vi "KsPS_Control.vi"() -> ()   [LabVIEW 2015]
doc: "This VI tool is designed to control Agilent/Keysight N67xx series power supply mainframes.\n\nFor support contact: Aldrin Albano, J54147"
uses:
  <vilib>/Utility/sysdir.llb/System Directory Type.ctl
  <vilib>/Utility/file.llb/Read Delimited Spreadsheet (string).vi
  <vilib>/Utility/file.llb/Write Delimited Spreadsheet (string).vi
  <instrlib>/Agilent N6700 Series/Agilent N6700 Series.lvlib
panel:
  in  "Tab Control":enum32{"Main", "Config", "Status"}(tab)
  out "OVP1":dbl format="%.3f"
  out "OVP4":dbl format="%.3f"
  out "OVP3":dbl format="%.3f"
  out "OVP2":dbl format="%.3f"
  out "State":string="Close GUI"
  out "Revision":string
  out "Ch4-I":dbl format="%.3f"
  out "Ch4-V":dbl format="%.3f"
  out "Ch3-I":dbl format="%.3f"
  out "Ch3-V":dbl format="%.3f"
  out "Ch2-I":dbl format="%.3f"
  out "Ch2-V":dbl format="%.3f"
  out "Ch1-V":dbl format="%.3f"
  out "Ch1-I":dbl format="%.3f"
  in  "Auto On/Off":bool
  in  "Auto Query":bool
  in  "Lock":bool=TRUE
  in  "Rvs Pwr Down":bool=TRUE
  in  "On/Off":bool
  in  "PS Settings":string[][](table)
  in  "Config_PATH":path
  in  "Load":bool
  in  "Query":bool
  in  "Save":bool
  in  "ResetOVP":bool
  in  "Qry Intrvl (ms)":u32=5000
  out "Open VISA Sessions":refnum<visa-resource-name>[](array[refnum])
  out "INI PATH":path
  out "Error Out":errorcluster
  # "OVP"
  # "OVP"
  # "OVP"
  # "OVP"
  # "V"
  # "A"
  # "V"
  # "A"
  # "V"
  # "A"
  # "V"
  # "A"
  # "Keysight N6700 Series PS Control Utility"
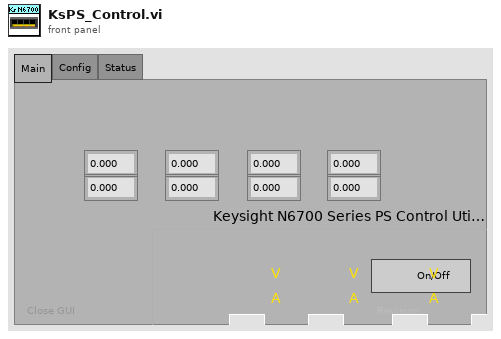
[diagram p1: front panel]
types:
  T1 = cluster{"PS Settings":string[][], "Config_PATH":path, "INI_PATH":path, "Open Sessions":refnum<visa-resource-name>[], "This VI":refnum<vi>, "VI Name":string}
  T2 = typedef "System Directory Type.ctl" = i32
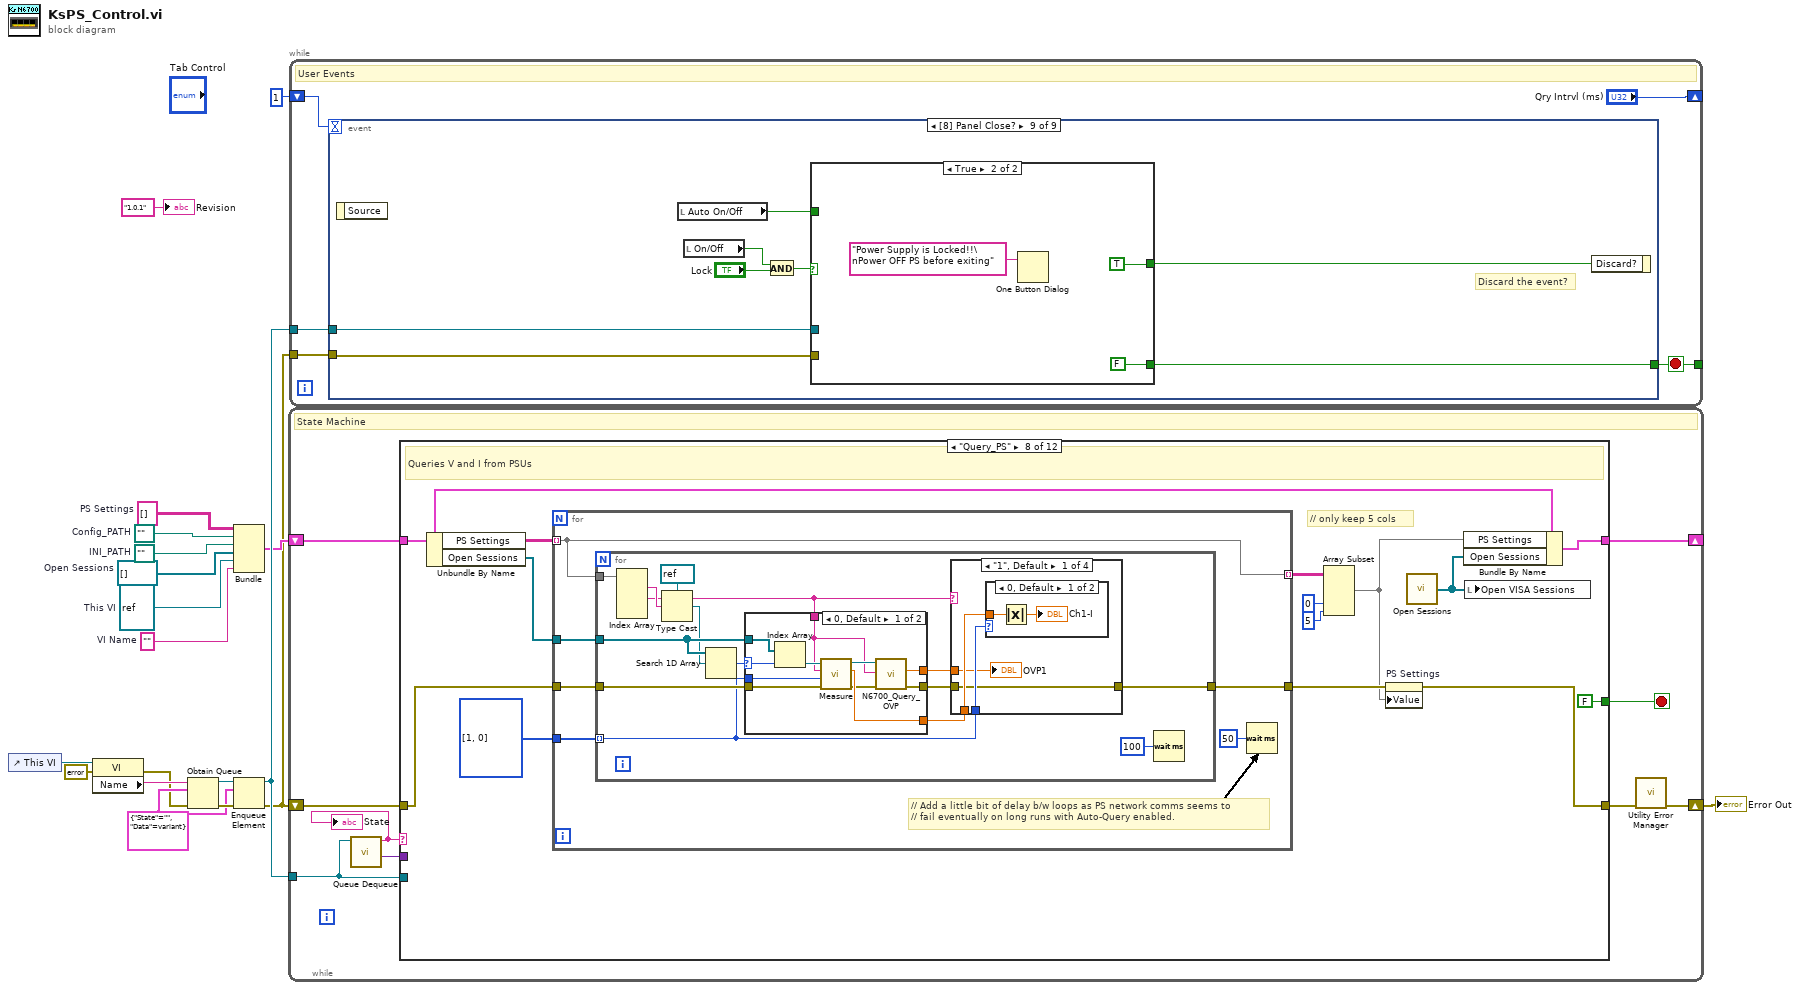
[diagram p0: block diagram]
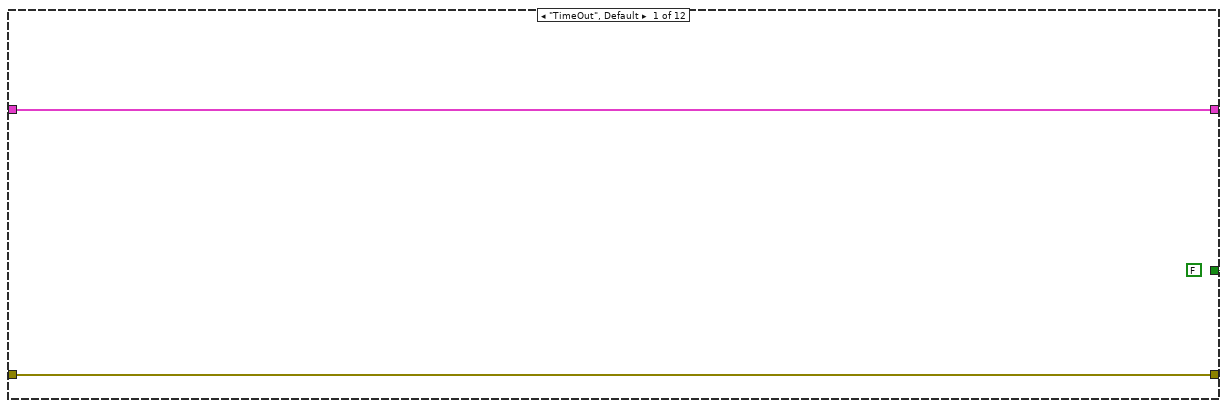
[diagram p2: hidden frame]
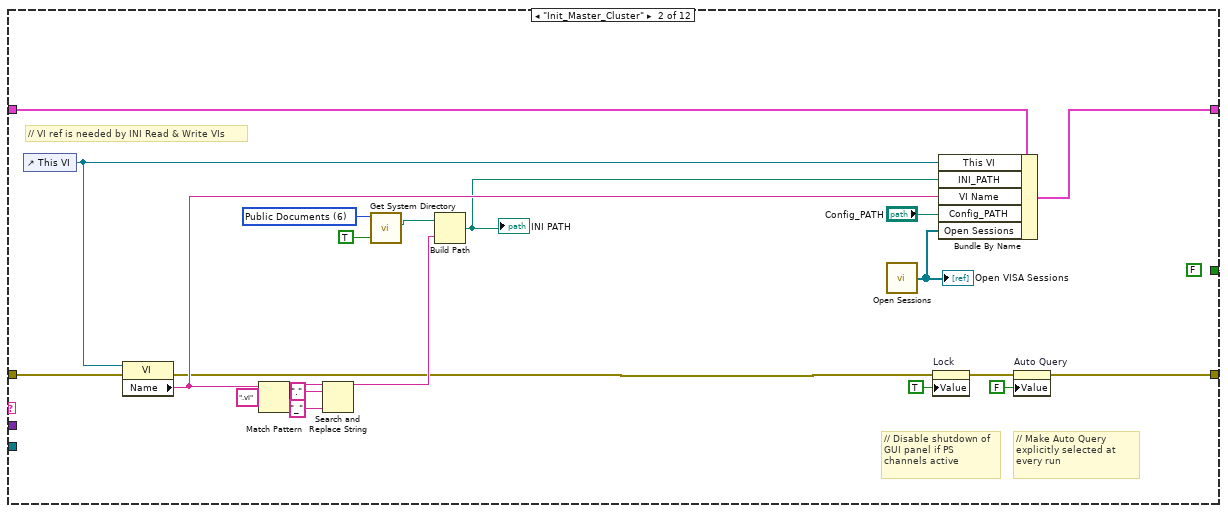
[diagram p3: hidden frame]
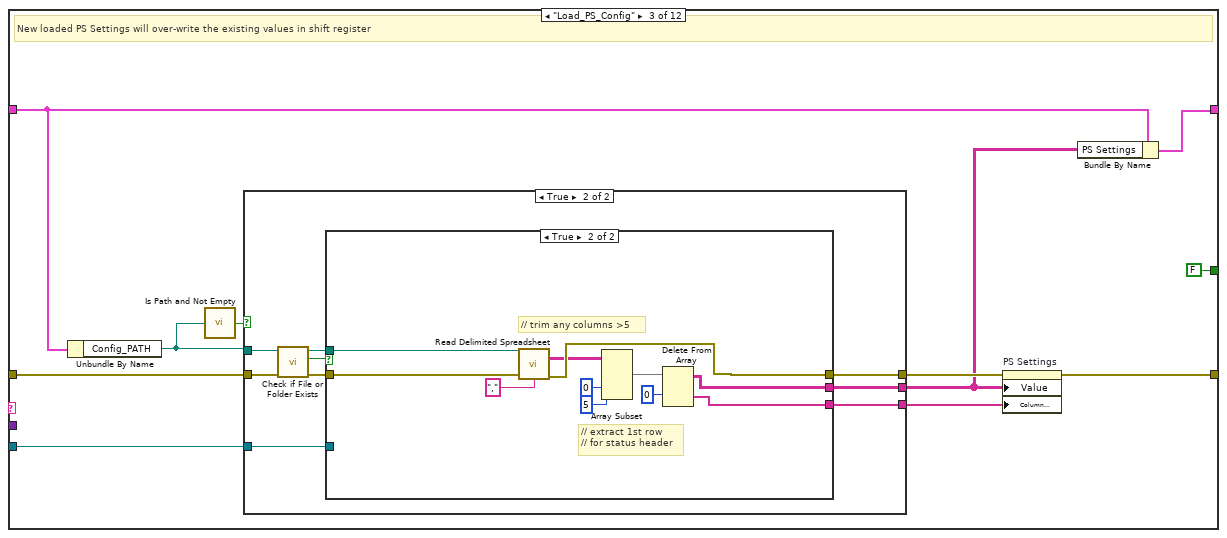
[diagram p4: hidden frame]
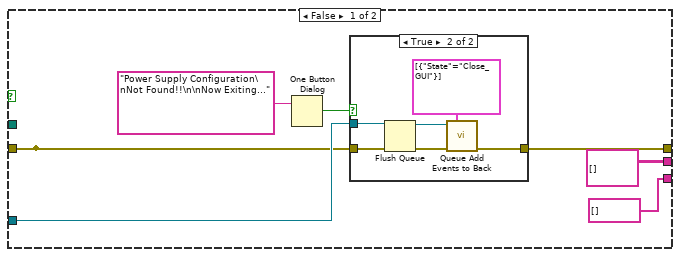
[diagram p5: hidden frame]
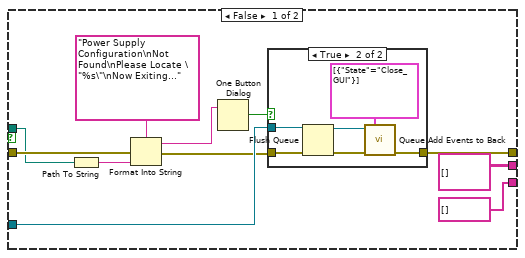
[diagram p7: hidden frame]
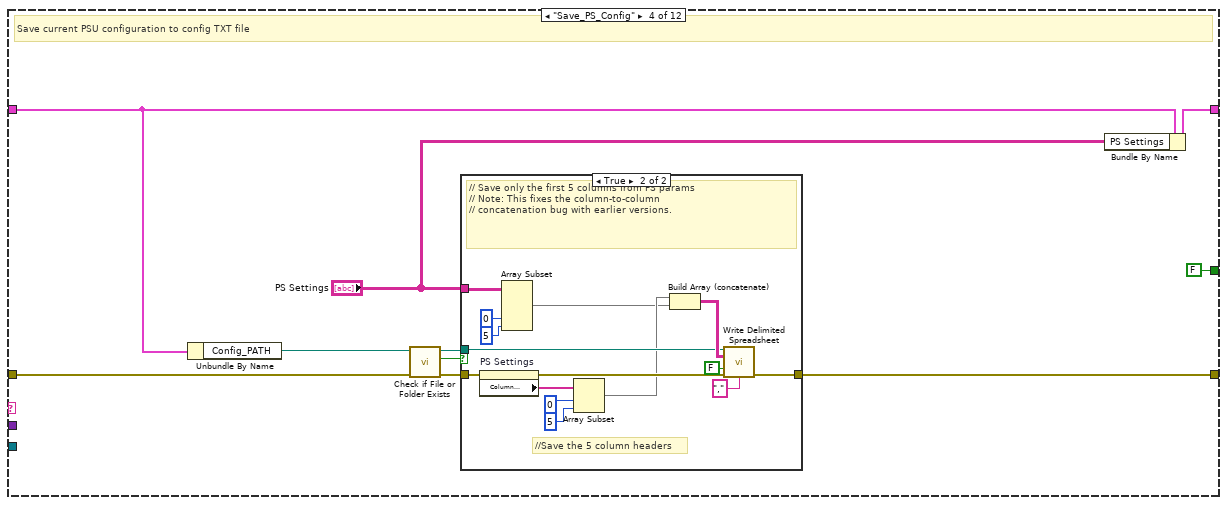
[diagram p9: hidden frame]
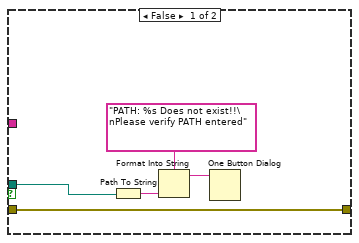
[diagram p10: hidden frame]
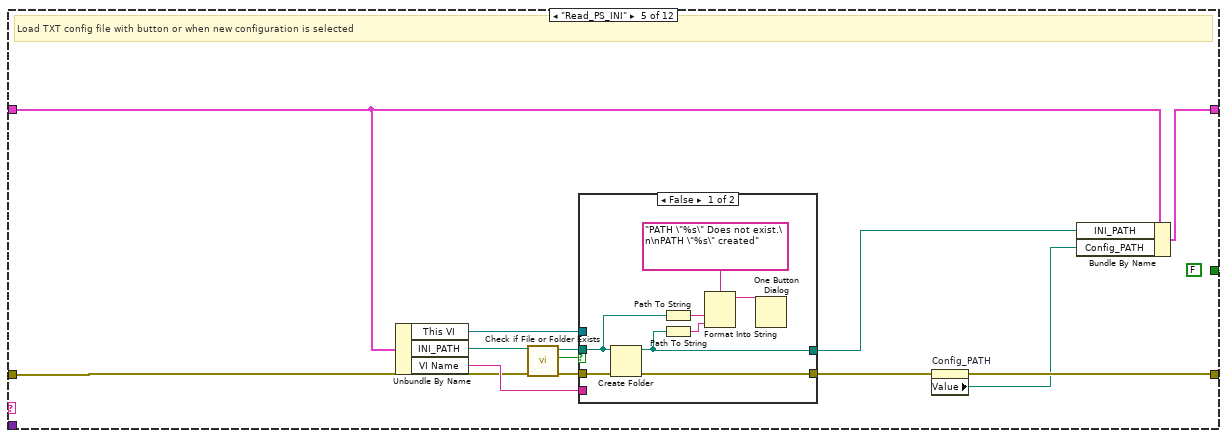
[diagram p11: hidden frame]
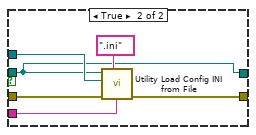
[diagram p12: hidden frame]
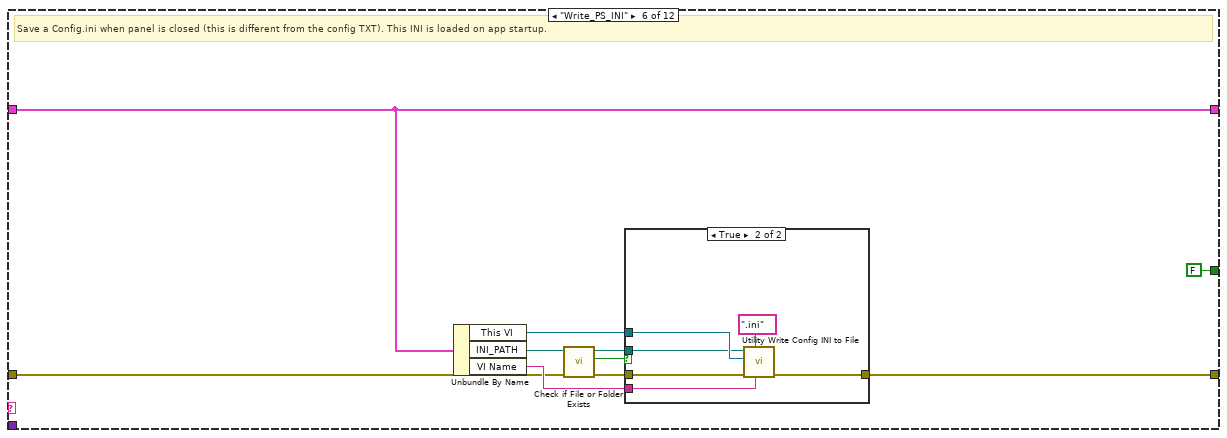
[diagram p13: hidden frame]
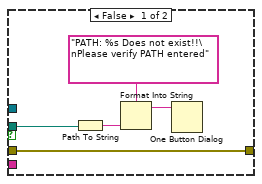
[diagram p14: hidden frame]
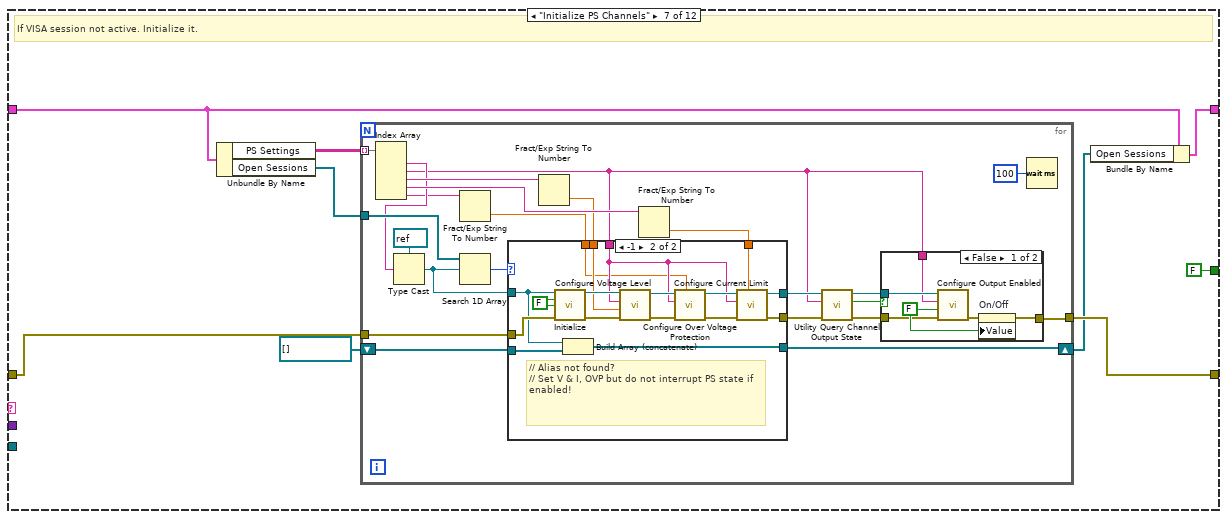
[diagram p15: hidden frame]
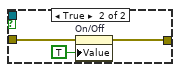
[diagram p16: hidden frame]
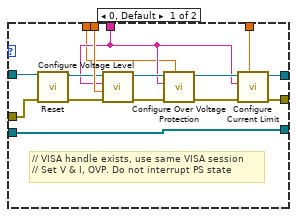
[diagram p17: hidden frame]
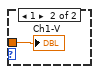
[diagram p18: hidden frame]
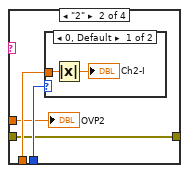
[diagram p19: hidden frame]
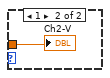
[diagram p20: hidden frame]
diagram:
  w2 = ""  # VI Name
  w3 = refnum<visa-resource-name>[] []  # Open Sessions
  w4 = refnum<vi> refnum  # This VI
  w6 = string[][] []  # PS Settings
  w7 = path ""  # INI_PATH
  w8 = path ""  # Config_PATH
  w17 = cluster{"State":string, "Data":variant} {"State"="", "Data"=variant} ("Cluster")
  n1 = control-ref of="This VI"() -> (w1:refnum<vi>)
  n2 = property class="VI"(reference=w1, error in=errorcluster {"status"=FALSE, "code"=0, "source"=""} ("Error In")) -> (error out=w13:errorcluster, "Name"=w15:string)  [unwired: 1 out]
  n3 = Obtain Queue(name (unnamed)=w15, element data type=w17, error in (no error)=w13) -> (queue out=w18:refnum<queue>, error out=w19:errorcluster)  [unwired: 2 in, 1 out]
  n4 = Bundle("PS Settings"=w6, "Config_PATH"=w8, "INI_PATH"=w7, "Open Sessions"=w3, "This VI"=w4, "VI Name"=w2) -> (w9:T1)  [unwired: 1 in]
  n5 = Enqueue Element(queue=w18, element=w17, error in (no error)=w19) -> (queue out=w16:refnum<queue>, error out=w5:errorcluster)  [unwired: 1 in, 1 out]
  n6 = while {
    shift-right: [w28] -> w11
    shift-left: w5 -> [w25]
    shift-right: [w20] -> _
    shift-left: w9 -> [w24]
    tunnel: w16 -> [w21]
    stop <- w26 stop-if-true
    # "State Machine"
    n7 = call "Queue Dequeue.vi"("Queue In"=w21) -> ("Data"=w22:variant, "State"=w23:string)  [unwired: 8 in, 1 out]
    "State" <- w23
    n8 = case shown="\"Query_PS\"" w23 {
      tunnel: w25 -> [w30 w52 w59 w123 w155 w178 w196 w279 w342 w361 w377 w395]
      tunnel: [w30 w47 w56 w124 w147 w182 w201 w276 w345 w357 w380 w390] -> w27
      tunnel: w21 -> [_ _ w58 _ _ _ _ _ _ _ _ w397]
      tunnel: [FALSE FALSE FALSE FALSE FALSE FALSE FALSE FALSE FALSE FALSE FALSE TRUE] -> w26
      tunnel: w24 -> [w29 w50 w55 w117 w158 w180 w199 w278 w343 w356 w378 w393]
      tunnel: w22 -> [_ _ _ _ _ _ _ _ _ _ _ _]
      tunnel: [w29 w51 w61 w122 w157 w180 w198 w271 w343 w356 w378 w393] -> w20
      frame "TimeOut", Default {
        (unwired) FALSE
      }
      frame "Init_Master_Cluster" {
        w43 = T2 6 items=["User Home"=0, "User Desktop"=1, "User Documents"=2, "User Application Data"=3, "User Preferences"=4, "User Temporary"=5, "Public Documents"=6, "Public Application Data"=7, "Public Preferences"=8, "Public Cache"=13, "System Core Libraries"=9, "System Installed Libraries"=10, "Application Files"=11, "Boot Volume Root"=12] ("system directory type")
        (unwired) FALSE
        # "// Disable shutdown of GUI panel if PS channels active"
        # "// Make Auto Query explicitly selected at every run"
        # "// VI ref is needed by INI Read & Write VIs"
        n9 = control-ref of="This VI"() -> (w48:refnum<vi>)
        n10 = property class="VI"(reference=w48, error in=w52) -> (error out=w33:errorcluster, "Name"=w35:string)  [unwired: 1 out]
        n11 = Match Pattern(string=w35, regular expression=".vi") -> (before substring=w37:string)  [unwired: 1 in, 3 out]
        n12 = Search and Replace String(input string=w37, search string=".", replace string="_" ("replace string (\"\")")) -> (result string=w36:string)  [unwired: 5 in, 3 out]
        n13 = call <vilib>:"Get System Directory.vi"("create directory if not found? (F)"=TRUE, "system directory type"=w43) -> ("system directory"=w41:path)  [unwired: 9 in]
        n14 = Build Path(base path=w41, name or relative path=w36) -> (appended path=w34:path)
        "INI PATH" <- w34
        n15 = call <vilib>:"Open Sessions.vi"() -> ("Array of Refnums"=w49:refnum<visa-resource-name>[])  [unwired: 2 in]
        "Open VISA Sessions" <- w49
        n16 = property on="Lock" class="Bool (strict)"(error in=w33, "Value"=TRUE ("Lock")) -> (error out=w45:errorcluster)  [unwired: 1 in, 1 out]
        n17 = Bundle By Name(cluster=w50, "This VI"=w48, "INI_PATH"=w34, "VI Name"=w35, "Config_PATH"="Config_PATH", "Open Sessions"=w49) -> (w51:T1)
        n18 = property on="Auto Query" class="Bool (strict)"(error in=w45, "Value"=FALSE ("Auto Query")) -> (error out=w47:errorcluster)  [unwired: 1 in, 1 out]
      }
      frame "Load_PS_Config" {
        # "New loaded PS Settings will over-write the existing values in shift register"
        n19 = Unbundle By Name(w55) -> ("Config_PATH"=w54:path)
        n20 = call <vilib>:"Is Path and Not Empty.vi"("path"=w54) -> ("Is Path and Not Empty?"=w57:bool)  [unwired: 4 in]
        n21 = case shown="True" w57 {
          tunnel: [w66 w86] -> w64
          tunnel: [string[] [] ("all rows") w85] -> w63
          tunnel: [string[][] [] w84] -> w60
          tunnel: w58 -> [w68 w83]
          tunnel: w59 -> [w66 w81]
          tunnel: w54 -> [_ w78]
          frame False {
            n22 = One Button Dialog(message="Power Supply Configuration\nNot Found!!\n\nNow Exiting...") -> (true=w67:bool)  [unwired: 1 in]
            n23 = case shown="True" w67 {
              tunnel: w68 -> [_ w75]
              tunnel: w66 -> [w71 w73]
              tunnel: [w71 w76] -> _
              frame False {
              }
              frame True {
                n24 = Flush Queue(queue=w75, error in (no error)=w73) -> (queue out=w74:refnum<queue>, error out=w72:errorcluster)  [unwired: 1 out]
                n25 = call "Queue Add Events to Back.vi"("Queue In"=w74, "State Array"=cluster{"State":string}[] [{"State"="Close_GUI"}], "Error In"=w72) -> ("Error Out"=w76:errorcluster)  [unwired: 11 in, 1 out]
              }
            }
          }
          frame True {
            n26 = call <vilib>:"Check if File or Folder Exists.vi"("error in (no error)"=w81, "path"=w78) -> ("error out"=w80:errorcluster, "file or folder exists?"=w79:bool, "dup path"=w82:path)  [unwired: 7 in]
            n27 = case shown="True" w79 {
              tunnel: [w93 w115] -> w86
              tunnel: [string[] [] ("all rows") w114] -> w85
              tunnel: [string[][] [] w113] -> w84
              tunnel: w80 -> [w90 w112]
              tunnel: w82 -> [w88 w111]
              tunnel: w83 -> [w95 _]
              frame False {
                n28 = Path To String(path=w88) -> (string=w87:string)
                n29 = Format Into String(format string="Power Supply Configuration\nNot Found\nPlease Locate \"%s\"\nNow Exiting..." ("message"), error in=w90, w87) -> (resulting string=w91:string, error out=w89:errorcluster)  [unwired: 1 in]
                n30 = One Button Dialog(message=w91) -> (true=w94:bool)  [unwired: 1 in]
                n31 = case shown="True" w94 {
                  tunnel: w95 -> [_ w102]
                  tunnel: w89 -> [w98 w100]
                  tunnel: [w98 w103] -> w93
                  frame False {
                  }
                  frame True {
                    n32 = Flush Queue(queue=w102, error in (no error)=w100) -> (queue out=w101:refnum<queue>, error out=w99:errorcluster)  [unwired: 1 out]
                    n33 = call "Queue Add Events to Back.vi"("Queue In"=w101, "State Array"=cluster{"State":string}[] [{"State"="Close_GUI"}], "Error In"=w99) -> ("Error Out"=w103:errorcluster)  [unwired: 11 in, 1 out]
                  }
                }
              }
              frame True {
                # "// trim any columns >5"
                # "// extract 1st row\n// for status header"
                n34 = call-poly <vilib>:"Read Delimited Spreadsheet.vi"("file path (dialog if empty)"=w111, "error in (no error)"=w112, "delimiter (\\t)"="," ("delimiter (\\t)")) -> ("all rows"=w106:string[][], "error out"=w115:errorcluster)  [unwired: 7 in, 4 out]
                n35 = Array Subset(array=w106, index (col)=0 ("index"), length (col)=5 ("length")) -> (w105:string[][])  [unwired: 2 in]
                n36 = Delete From Array(array=w105, index (row)=0) -> (deleted portion=w114:string[], array with subset deleted=w113:string[][])  [unwired: 2 in]
              }
            }
          }
        }
        n37 = property on="PS Settings" class="Tbl (strict)"(error in=w64, "Value"=w60, "Column Headers[]"=w63) -> (error out=w56:errorcluster)  [unwired: 1 in, 1 out]
        n38 = Bundle By Name(cluster=w55, "PS Settings"=w60) -> (w61:T1)
      }
      frame "Save_PS_Config" {
        # "Save current PSU configuration to config TXT file"
        n39 = Unbundle By Name(w117) -> ("Config_PATH"=w116:path)
        n40 = call <vilib>:"Check if File or Folder Exists.vi"("error in (no error)"=w123, "path"=w116) -> ("error out"=w120:errorcluster, "file or folder exists?"=w118:bool, "dup path"=w119:path)  [unwired: 7 in]
        n41 = case shown="True" w118 {
          tunnel: [w130 w142] -> w124
          tunnel: "PS Settings" -> [_ w134]
          tunnel: w119 -> [w126 w140]
          tunnel: w120 -> [w130 w133]
          frame False {
            n42 = Path To String(path=w126) -> (string=w128:string)
            n43 = Format Into String(format string="PATH: %s Does not exist!!\nPlease verify PATH entered", w128) -> (resulting string=w127:string)  [unwired: 2 in, 1 out]
            n44 = One Button Dialog(message=w127) -> ()  [unwired: 1 in, 1 out]
          }
          frame True {
            # "//Save the 5 column headers"
            # "// Save only the first 5 columns from PS params\n// Note: This fixes the column-to-column\n// concatenation bug with earlier versions."
            n45 = property on="PS Settings" class="Tbl (strict)"(error in=w133) -> (error out=w143:errorcluster, "Column Headers[]"=w137:string[])  [unwired: 1 in, 1 out]
            n46 = Array Subset(array=w134, index (col)=0 ("index"), length (col)=5 ("length")) -> (w131:string[][])  [unwired: 2 in]
            n47 = Array Subset(array=w137, index=0, length=5) -> (w132:string[])
            n48 = Build Array (concatenate)(w132, w131) -> (w141:string[][])
            n49 = call-poly <vilib>:"Write Delimited Spreadsheet.vi"("file path (dialog if empty)"=w140, "2D data"=w141, "append to file? (F)"=FALSE, "error in (no error)"=w143, "delimiter (\\t)"="," ("delimiter (\\t)")) -> ("error out"=w142:errorcluster)  [unwired: 9 in, 1 out]
          }
        }
        n50 = Bundle By Name(cluster=w117, "PS Settings"="PS Settings") -> (w122:T1)
      }
      frame "Read_PS_INI" {
        (unwired) FALSE
        # "Load TXT config file with button or when new configuration is selected"
        n51 = Unbundle By Name(w158) -> ("This VI"=w150:refnum<vi>, "INI_PATH"=w153:path, "VI Name"=w156:string)
        n52 = call <vilib>:"Check if File or Folder Exists.vi"("error in (no error)"=w155, "path"=w153) -> ("error out"=w154:errorcluster, "file or folder exists?"=w151:bool, "dup path"=w152:path)  [unwired: 7 in]
        n53 = case shown="False" w151 {
          tunnel: [w164 w171] -> w148
          tunnel: w154 -> [w164 w170]
          tunnel: w152 -> [w162 w167]
          tunnel: w150 -> [_ w169]
          tunnel: [w160 w167] -> w149
          tunnel: w156 -> [_ w168]
          frame False {
            n54 = Create Folder(path (use dialog)=w162, error in=w164) -> (created path=w160:path)  [unwired: 1 in, 2 out]
            n55 = Path To String(path=w162) -> (string=w163:string)
            n56 = Path To String(path=w160) -> (string=w161:string)
            n57 = Format Into String(format string="PATH \"%s\" Does not exist.\n\nPATH \"%s\" created", w163, w161) -> (resulting string=w165:string)  [unwired: 2 in, 1 out]
            n58 = One Button Dialog(message=w165) -> ()  [unwired: 1 in, 1 out]
          }
          frame True {
            n59 = call "Utility Load Config INI from File.vi"("File Name"=w168, "File Type"=".ini", "Error In"=w170, "reference"=w169, "Path In"=w167) -> ("Error Out"=w171:errorcluster)  [unwired: 5 in, 1 out]
          }
        }
        n60 = property on="Config_PATH" class="Path"(error in=w148) -> (error out=w147:errorcluster, "Value"=w146:path)  [unwired: 1 in, 1 out]
        n61 = Bundle By Name(cluster=w158, "INI_PATH"=w149, "Config_PATH"=w146) -> (w157:T1)
      }
      frame "Write_PS_INI" {
        # "Save a Config.ini when panel is closed (this is different from the config TXT). This INI is loaded on app startup."
        n62 = Unbundle By Name(w180) -> ("This VI"=w173:refnum<vi>, "INI_PATH"=w175:path, "VI Name"=w179:string)
        n63 = call <vilib>:"Check if File or Folder Exists.vi"("error in (no error)"=w178, "path"=w175) -> ("error out"=w177:errorcluster, "file or folder exists?"=w176:bool, "dup path"=w174:path)  [unwired: 7 in]
        n64 = case shown="True" w176 {
          tunnel: w177 -> [w187 w193]
          tunnel: [w187 w192] -> w182
          tunnel: w174 -> [w183 w188]
          tunnel: w173 -> [_ w190]
          tunnel: w179 -> [_ w189]
          frame False {
            n65 = Path To String(path=w183) -> (string=w185:string)
            n66 = Format Into String(format string="PATH: %s Does not exist!!\nPlease verify PATH entered", w185) -> (resulting string=w184:string)  [unwired: 2 in, 1 out]
            n67 = One Button Dialog(message=w184) -> ()  [unwired: 1 in, 1 out]
          }
          frame True {
            n68 = call "Utility Write Config INI to File.vi"("File Name"=w189, "File Type"=".ini", "Error In"=w193, "reference"=w190, "Path In"=w188) -> ("Error Out"=w192:errorcluster)  [unwired: 5 in, 1 out]
          }
        }
      }
      frame "Initialize PS Channels" {
        # "If VISA session not active. Initialize it."
        n69 = Unbundle By Name(w199) -> ("PS Settings"=w202:string[][], "Open Sessions"=w194:refnum<visa-resource-name>[])
        n70 = for {
          tunnel: w202 -> [w224] mode=indexing
          shift-right: [w222] -> w197
          shift-left: refnum<visa-resource-name>[] [] -> [w225]
          tunnel: [w208] -> w201
          tunnel: w196 -> [w216]
          tunnel: w194 -> [w215]
          n71 = Index Array(array=w224) -> (element #1=w214:string, element #2=w206:string, element #3=w220:string, element #4=w219:string, element #5=w204:string)  [unwired: 5 in]
          n72 = Type Cast(type=refnum<visa-resource-name> refnum ("VISA resource name"), x=w214) -> (*(type *) &x=w212:refnum<visa-resource-name>)
          n73 = Fract/Exp String To Number(string=w204) -> (number=w203:dbl)  [unwired: 3 in, 1 out]
          n74 = Search 1D Array(1D array=w215, element=w212) -> (index of element=w221:i32)  [unwired: 1 in]
          n75 = Fract/Exp String To Number(string=w220) -> (number=w217:dbl)  [unwired: 3 in, 1 out]
          n76 = Fract/Exp String To Number(string=w219) -> (number=w218:dbl)  [unwired: 3 in, 1 out]
          n77 = case shown="-1" w221 {
            tunnel: [w249 w266] -> w222
            tunnel: w225 -> [w249 w265]
            tunnel: [w247 w252] -> w210
            tunnel: w216 -> [w238 w264]
            tunnel: w212 -> [w240 w260]
            tunnel: w218 -> [w248 w261]
            tunnel: w217 -> [w242 w254]
            tunnel: w206 -> [w236 w253]
            tunnel: [w241 w251] -> w211
            tunnel: w203 -> [w235 w250]
            frame 0, Default {
              # "// VISA handle exists, use same VISA session\n// Set V & I, OVP. Do not interrupt PS state"
              n78 = call <instrlib>:"Reset.vi"("VISA resource name"=w240, "error in (no error)"=w238) -> ("VISA resource name out"=w239:refnum<visa-resource-name>, "error out"=w237:errorcluster)  [unwired: 12 in]
              n79 = call <instrlib>:"Configure Voltage Level.vi"("error in (no error)"=w237, "Level  (0.0 volts)"=w242, "Channel Name (1)"=w236, "VISA resource name"=w239) -> ("error out"=w246:errorcluster, "VISA resource name out"=w244:refnum<visa-resource-name>)  [unwired: 6 in]
              n80 = call <instrlib>:"Configure Over Voltage Protection.vi"("Limit (0.0 volts)"=w235, "error in (no error)"=w246, "Channel Name (1)"=w236, "VISA resource name"=w244) -> ("error out"=w245:errorcluster, "VISA resource name out"=w243:refnum<visa-resource-name>)  [unwired: 6 in]
              n81 = call <instrlib>:"Configure Current Limit.vi"("Limit (0.0 amps)"=w248, "error in (no error)"=w245, "Channel Name (1)"=w236, "VISA resource name"=w243) -> ("error out"=w247:errorcluster, "VISA resource name out"=w241:refnum<visa-resource-name>)  [unwired: 6 in]
            }
            frame -1 {
              w259 = FALSE ("ID Query? (T: Yes)")
              # "// Alias not found?\n// Set V & I, OVP but do not interrupt PS state if enabled!"
              n82 = call <instrlib>:"Initialize.vi"("VISA resource name"=w260, "ID Query? (T: Yes)"=w259, "Reset? (T: Yes)"=w259, "error in (no error)"=w264) -> ("VISA resource name out"=w262:refnum<visa-resource-name>, "error out"=w263:errorcluster)  [unwired: 10 in]
              n83 = Build Array (concatenate)(w260, w265) -> (w266:refnum<visa-resource-name>[])
              n84 = call <instrlib>:"Configure Voltage Level.vi"("error in (no error)"=w263, "Level  (0.0 volts)"=w254, "Channel Name (1)"=w253, "VISA resource name"=w262) -> ("error out"=w258:errorcluster, "VISA resource name out"=w256:refnum<visa-resource-name>)  [unwired: 6 in]
              n85 = call <instrlib>:"Configure Over Voltage Protection.vi"("Limit (0.0 volts)"=w250, "error in (no error)"=w258, "Channel Name (1)"=w253, "VISA resource name"=w256) -> ("error out"=w257:errorcluster, "VISA resource name out"=w255:refnum<visa-resource-name>)  [unwired: 6 in]
              n86 = call <instrlib>:"Configure Current Limit.vi"("Limit (0.0 amps)"=w261, "error in (no error)"=w257, "Channel Name (1)"=w253, "VISA resource name"=w255) -> ("error out"=w252:errorcluster, "VISA resource name out"=w251:refnum<visa-resource-name>)  [unwired: 6 in]
            }
          }
          n87 = call "Utility Query Channel Output State.vi"("error in (no error)"=w210, "Channel Name (1)"=w206, "VISA resource name"=w211) -> ("error out"=w209:errorcluster, "In State"=w205:bool, "VISA resource name out"=w207:refnum<visa-resource-name>)  [unwired: 6 in]
          n88 = case shown="False" w205 {
            tunnel: [w230 w234] -> w208
            tunnel: w209 -> [w228 w232]
            tunnel: w207 -> [w227 _]
            tunnel: w206 -> [w226 _]
            frame False {
              w229 = FALSE ("Enable Output (False)")
              n89 = call <instrlib>:"Configure Output Enabled.vi"("error in (no error)"=w228, "Enable Output (False)"=w229, "Channel Name (1)"=w226, "VISA resource name"=w227) -> ("error out"=w231:errorcluster)  [unwired: 6 in, 1 out]
              n90 = property on="On/Off" class="Bool (strict)"(error in=w231, "Value"=w229) -> (error out=w230:errorcluster)  [unwired: 1 in, 1 out]
            }
            frame True {
              n91 = property on="On/Off" class="Bool (strict)"(error in=w232, "Value"=TRUE ("On/Off")) -> (error out=w234:errorcluster)  [unwired: 1 in, 1 out]
            }
          }
          n92 = Wait (ms)(milliseconds to wait=u32 100) -> ()  [unwired: 1 out]
        }
        n93 = Bundle By Name(cluster=w199, "Open Sessions"=w197) -> (w198:T1)
      }
      frame "Query_PS" {
        w268 = i32[] [1, 0] items=["Voltage"=1, "Current"=0]
        # "// only keep 5 cols"
        # "Queries V and I from PSUs"
        n94 = Unbundle By Name(w278) -> ("PS Settings"=w275:string[][], "Open Sessions"=w269:refnum<visa-resource-name>[])
        n95 = for {
          tunnel: w279 -> [w286]
          tunnel: [w285] -> w280
          tunnel: w275 -> [w284] mode=indexing
          tunnel: [w284] -> w272 mode=indexing
          tunnel: w269 -> [w282]
          tunnel: w268 -> [w281]
          # "// Add a little bit of delay b/w loops as PS network comms seems to\n// fail eventually on long runs with Auto-Query enabled."
          n96 = for {
            tunnel: w281 -> [w292] mode=indexing
            tunnel: w286 -> [w297]
            tunnel: [w287] -> w285
            tunnel: w284 -> [w300]
            tunnel: w282 -> [w294]
            n97 = Index Array(array=w300) -> (element #1=w298:string, element #2=w291:string)  [unwired: 4 in, 2 out]
            n98 = Type Cast(type=refnum<visa-resource-name> refnum ("VISA resource name"), x=w298) -> (*(type *) &x=w290:refnum<visa-resource-name>)
            n99 = Search 1D Array(1D array=w294, element=w290) -> (index of element=w295:i32)  [unwired: 1 in]
            n100 = case shown="0, Default" w295 {
              selector: w295 -> [w336 _]
              tunnel: w292 -> [w339 _]
              tunnel: [w332 w341] -> w288
              tunnel: w291 -> [w330 _]
              tunnel: [w338 w340] -> w293
              tunnel: w297 -> [w337 w341]
              tunnel: w294 -> [w335 _]
              tunnel: [w329 w340] -> w289
              frame 0, Default {
                n101 = Index Array(array=w335, index=w336) -> (element=w334:refnum<visa-resource-name>)
                n102 = call <instrlib>:"Measure.vi"("error in (no error)"=w337, "Measurement Type (1: Voltage)"=w339, "Channel Name (1)"=w330, "VISA resource name"=w334) -> ("error out"=w333:errorcluster, "Measurement"=w338:dbl, "VISA resource name out"=w331:refnum<visa-resource-name>)  [unwired: 5 in]
                n103 = call "N6700_Query_OVP.vi"("error in (no error)"=w333, "Channel Name (1)"=w330, "VISA resource name"=w331) -> ("error out"=w332:errorcluster, "Measurement"=w329:dbl)  [unwired: 6 in, 1 out]
              }
              frame -1 {
                w340 = 0.0 ("Measurement")
              }
            }
            n104 = case shown="\"1\", Default" w291 {
              tunnel: w293 -> [w304 w311 w318 w325]
              tunnel: w292 -> [w303 w310 w317 w324]
              tunnel: w289 -> [w302 w309 w316 w323]
              tunnel: w288 -> [w301 w308 w315 w322]
              tunnel: [w301 w308 w315 w322] -> w287
              frame "1", Default {
                n105 = case shown="0, Default" w303 {
                  tunnel: w304 -> [w305 w307]
                  frame 0, Default {
                    n106 = Absolute Value(x=w305) -> (abs(x)=→"Ch1-I":dbl)
                  }
                  frame 1 {
                    "Ch1-V" <- w307
                  }
                }
                "OVP1" <- w302
              }
              frame "2" {
                n107 = case shown="0, Default" w310 {
                  tunnel: w311 -> [w313 w314]
                  frame 0, Default {
                    n108 = Absolute Value(x=w313) -> (abs(x)=→"Ch2-I":dbl)
                  }
                  frame 1 {
                    "Ch2-V" <- w314
                  }
                }
                "OVP2" <- w309
              }
              frame "3" {
                n109 = case shown="0, Default" w317 {
                  tunnel: w318 -> [w319 w321]
                  frame 0, Default {
                    n110 = Absolute Value(x=w319) -> (abs(x)=→"Ch3-I":dbl)
                  }
                  frame 1 {
                    "Ch3-V" <- w321
                  }
                }
                "OVP3" <- w316
              }
              frame "4" {
                n111 = case shown="0, Default" w324 {
                  tunnel: w325 -> [w326 w328]
                  frame 0, Default {
                    n112 = Absolute Value(x=w326) -> (abs(x)=→"Ch4-I":dbl)
                  }
                  frame 1 {
                    "Ch4-V" <- w328
                  }
                }
                "OVP4" <- w323
              }
            }
            n113 = Wait (ms)(milliseconds to wait=u32 100) -> ()  [unwired: 1 out]
          }
          n114 = Wait (ms)(milliseconds to wait=u32 50) -> ()  [unwired: 1 out]
        }
        n115 = Array Subset(array=w272, index (col)=0 ("index"), length (col)=5 ("length")) -> (w267:string[][])  [unwired: 2 in]
        n116 = property on="PS Settings" class="Tbl (strict)"(error in=w280, "Value"=w267) -> (error out=w276:errorcluster)  [unwired: 1 in, 1 out]
        n117 = call <vilib>:"Open Sessions.vi"() -> ("Array of Refnums"=w270:refnum<visa-resource-name>[])  [unwired: 2 in]
        n118 = Bundle By Name(cluster=w278, "PS Settings"=w267, "Open Sessions"=w270) -> (w271:T1)
        n119 = local write "Open VISA Sessions"(w270) -> ()
      }
      frame "PS_On" {
        n120 = Unbundle By Name(w343) -> ("PS Settings"=w346:string[][])
        n121 = for {
          tunnel: w346 -> [w354] mode=indexing
          tunnel: [w355] -> w345
          tunnel: w342 -> [w347]
          n122 = Index Array(array=w354) -> (element #1=w349:string, element #2=w351:string)  [unwired: 4 in, 2 out]
          n123 = Type Cast(type=refnum<visa-resource-name> refnum ("VISA resource name"), x=w349) -> (*(type *) &x=w348:refnum<visa-resource-name>)
          n124 = call <instrlib>:"Configure Output Enabled.vi"("error in (no error)"=w347, "Enable Output (False)"=TRUE, "Channel Name (1)"=w351, "VISA resource name"=w348) -> ("error out"=w355:errorcluster)  [unwired: 6 in, 1 out]
          n125 = Wait (ms)(milliseconds to wait=u32 10) -> ()  [unwired: 1 out]
        }
      }
      frame "PS_Off" {
        n126 = Unbundle By Name(w356) -> ("PS Settings"=w360:string[][])
        n127 = Transpose 2D Array(2D array=w360) -> (transposed array=w365:string[][])
        n128 = for {
          tunnel: w365 -> [w367] mode=indexing
          tunnel: [w366] -> w363 mode=indexing
          n129 = Reverse 1D Array(array=w367) -> (reversed array=w366:string[])
        }
        n130 = Transpose 2D Array(2D array=w363) -> (transposed array=w364:string[][])
        n131 = Select(t=w364, s="Rvs Pwr Down", f=w360) -> (s? t:f=w362:string[][])
        n132 = for {
          tunnel: w362 -> [w373] mode=indexing
          tunnel: [w375] -> w357
          tunnel: w361 -> [w369]
          n133 = Index Array(array=w373) -> (element #1=w374:string, element #2=w371:string)  [unwired: 4 in, 2 out]
          n134 = Type Cast(type=refnum<visa-resource-name> refnum ("VISA resource name"), x=w374) -> (*(type *) &x=w376:refnum<visa-resource-name>)
          n135 = call <instrlib>:"Configure Output Enabled.vi"("error in (no error)"=w369, "Enable Output (False)"=FALSE, "Channel Name (1)"=w371, "VISA resource name"=w376) -> ("error out"=w375:errorcluster)  [unwired: 6 in, 1 out]
          n136 = Wait (ms)(milliseconds to wait=u32 10) -> ()  [unwired: 1 out]
        }
      }
      frame "Reset_OVP" {
        n137 = Unbundle By Name(w378) -> ("PS Settings"=w381:string[][])
        n138 = for {
          tunnel: w381 -> [w389] mode=indexing
          tunnel: [w384] -> w380
          tunnel: w377 -> [w385]
          n139 = Index Array(array=w389) -> (element #1=w386:string, element #2=w382:string)  [unwired: 4 in, 2 out]
          n140 = Type Cast(type=refnum<visa-resource-name> refnum ("VISA resource name"), x=w386) -> (*(type *) &x=w383:refnum<visa-resource-name>)
          n141 = call <instrlib>:"Reset Output Protection.vi"("error in (no error)"=w385, "Channel Name (1)"=w382, "VISA resource name"=w383) -> ("error out"=w384:errorcluster)  [unwired: 7 in, 1 out]
          n142 = Wait (ms)(milliseconds to wait=u32 50) -> ()  [unwired: 1 out]
        }
      }
      frame "Close_GUI" {
        # "Empty & close queue. Close VISA sessions."
        n143 = Unbundle By Name(w393) -> ("Open Sessions"=w392:refnum<visa-resource-name>[])
        n144 = for {
          tunnel: w392 -> [w403] mode=indexing
          tunnel: w395 -> [w406]
          tunnel: [w405] -> w394
          n145 = Type Cast(type=refnum<visa-resource-name> refnum ("VISA resource name"), x=w403) -> (*(type *) &x=w402:refnum<visa-resource-name>)
          n146 = call <instrlib>:"Close.vi"("VISA resource name"=w402, "error in (no error)"=w406) -> ("error out"=w405:errorcluster)  [unwired: 13 in]
        }
        n147 = Flush Queue(queue=w397, error in (no error)=w394) -> (queue out=w396:refnum<queue>, error out=w398:errorcluster)  [unwired: 1 out]
        n148 = Release Queue(queue=w396, force destroy? (F)=TRUE, error in (no error)=w398) -> (error out=w391:errorcluster)  [unwired: 2 out]
        n149 = flat-sequence {
          tunnel: w391 -> [w401]
          tunnel: [w401] -> w390
          frame #0 {
            n150 = Stop() -> ()  [unwired: 1 in]
          }
        }
      }
    }
    n151 = call "Utility Error Manager.vi"("Error In"=w27) -> ("Error Out"=w28:errorcluster)  [unwired: 10 in]
  }
  "Error Out" <- w11
  n152 = while {
    tunnel: w16 -> [w411]
    tunnel: [w410] -> _
    shift-right: ["Qry Intrvl (ms)"] -> _
    shift-left: 1 -> [w409]
    tunnel: w5 -> [w407]
    stop <- w410 stop-if-true
    # "User Events"
    n153 = event shown="[8] Panel Close?" {
      selector: _ -> [_ _ _ _ _ _ _ _ _]
      dyn-events: _ -> [_ _ _ _ _ _ _ _ _]
      timeout: w409 -> [_ _ _ _ _ _ _ _ _]
      tunnel: w411 -> [w414 w429 w435 w440 w452 w459 w466 w473 w484]
      tunnel: [FALSE ("Abort?") FALSE ("Abort?") _ FALSE FALSE ("Discard?") FALSE ("Discard?") FALSE ("Discard?") FALSE ("Discard?") w480] -> w410
      tunnel: w407 -> [w412 _ w432 w439 w449 w456 w463 w471 w478]
      event Timeout {
        n154 = event-data() -> ()  [unwired: 1 in, 1 out]
        n155 = First Call?() -> (First Call?: T/F=w413:bool)
        n156 = case shown="True" w413 {
          tunnel: w414 -> [w418 w424]
          tunnel: w412 -> [w417 w422]
          frame True {
            n157 = case shown="False" "Auto On/Off" {
              tunnel: [cluster{"State":string}[] [{"State"="Init_Master_Cluster"}, {"State"="Read_PS_INI"}, {"State"="Load_PS_Config"}, {"State"="Initialize PS Channels"}] cluster{"State":string}[] [{"State"="Init_Master_Cluster"}, {"State"="Read_PS_INI"}, {"State"="Load_PS_Config"}, {"State"="Initialize PS Channels"}, {"State"="PS_On"}]] -> w419
              frame False {
              }
              frame True {
              }
            }
            n158 = call "Queue Add Events to Back.vi"("Queue In"=w418, "State Array"=w419, "Error In"=w417) -> ()  [unwired: 11 in, 2 out]
          }
          frame False {
            n159 = case shown="False" "Auto Query" {
              tunnel: w424 -> [_ w426]
              tunnel: w422 -> [_ w425]
              frame False {
              }
              frame True {
                n160 = call "Queue Add Events to Back.vi"("Queue In"=w426, "State Array"=cluster{"State":string}[] [{"State"="Query_PS"}], "Error In"=w425) -> ()  [unwired: 11 in, 2 out]
              }
            }
          }
        }
      }
      event Menu Selection (User) {
        n161 = event-data() -> ("ItemTag"=w431:string, "ItemPath"=w430:string)  [unwired: 1 in]
        n162 = case shown="Default" w430 {
          tunnel: w429 -> [_]
          tunnel: w431 -> [_]
          frame Default {
          }
        }
      }
      event "Config_PATH": Value Change {
        n163 = event-data() -> ("NewVal"=w434:path)  [unwired: 1 in]
        n164 = call <vilib>:"Is Path and Not Empty.vi"("path"=w434) -> ("Is Path and Not Empty?"=w433:bool)  [unwired: 4 in]
        n165 = case shown="True" w433 {
          tunnel: w435 -> [_ w438]
          tunnel: w432 -> [_ w436]
          frame False {
          }
          frame True {
            n166 = call "Queue Add Events to Back.vi"("Queue In"=w438, "State Array"=cluster{"State":string}[] [{"State"="Load_PS_Config"}, {"State"="Write_PS_INI"}], "Error In"=w436) -> ()  [unwired: 11 in, 2 out]
          }
        }
      }
      event "On/Off": Value Change {
        # "Initialize N67xx PSU with loaded configuration"
        n167 = event-data() -> ("NewVal"=w441:bool)  [unwired: 1 in]
        n168 = case shown="True" w441 {
          tunnel: w440 -> [w444 w447]
          tunnel: w439 -> [w443 w446]
          frame False {
            n169 = call "Queue Add Events to Back.vi"("Queue In"=w444, "State Array"=cluster{"State":string}[] [{"State"="PS_Off"}], "Error In"=w443) -> ()  [unwired: 11 in, 2 out]
          }
          frame True {
            n170 = call "Queue Add Events to Back.vi"("Queue In"=w447, "State Array"=cluster{"State":string}[] [{"State"="PS_On"}], "Error In"=w446) -> ()  [unwired: 11 in, 2 out]
          }
        }
      }
      event "Query": Value Change {
        n171 = event-data() -> ("NewVal"=w450:bool)  [unwired: 1 in]
        n172 = case shown="True" w450 {
          tunnel: w452 -> [_ w454]
          tunnel: w449 -> [_ w453]
          frame False {
          }
          frame True {
            n173 = call "Queue Add Events to Back.vi"("Queue In"=w454, "State Array"=cluster{"State":string}[] [{"State"="Query_PS"}], "Error In"=w453) -> ()  [unwired: 11 in, 2 out]
          }
        }
      }
      event "Load": Value Change {
        n174 = event-data() -> ("NewVal"=w457:bool)  [unwired: 1 in]
        n175 = case shown="True" w457 {
          tunnel: w459 -> [_ w461]
          tunnel: w456 -> [_ w460]
          frame False {
          }
          frame True {
            n176 = call "Queue Add Events to Back.vi"("Queue In"=w461, "State Array"=cluster{"State":string}[] [{"State"="Load_PS_Config"}, {"State"="Write_PS_INI"}], "Error In"=w460) -> ()  [unwired: 11 in, 2 out]
          }
        }
      }
      event "Save": Value Change {
        n177 = event-data() -> ("NewVal"=w464:bool)  [unwired: 1 in]
        n178 = case shown="True" w464 {
          tunnel: w466 -> [_ w468]
          tunnel: w463 -> [_ w467]
          frame False {
          }
          frame True {
            n179 = call "Queue Add Events to Back.vi"("Queue In"=w468, "State Array"=cluster{"State":string}[] [{"State"="Write_PS_INI"}, {"State"="Save_PS_Config"}], "Error In"=w467) -> ()  [unwired: 11 in, 2 out]
          }
        }
      }
      event "ResetOVP": Value Change {
        n180 = event-data() -> ("NewVal"=w470:bool)  [unwired: 1 in]
        n181 = case shown="True" w470 {
          tunnel: w473 -> [_ w475]
          tunnel: w471 -> [_ w474]
          frame False {
          }
          frame True {
            n182 = call "Queue Add Events to Back.vi"("Queue In"=w475, "State Array"=cluster{"State":string}[] [{"State"="Reset_OVP"}], "Error In"=w474) -> ()  [unwired: 11 in, 2 out]
          }
        }
      }
      event Panel Close? {
        # "Discard the event?"
        n183 = event-data() -> ()  [unwired: 1 in, 1 out]
        n184 = local read "Auto On/Off"() -> (w477:bool)
        n185 = local read "On/Off"() -> (w482:bool)
        n186 = And(x=w482, y="Lock") -> (x .and. y?=w481:bool)
        n187 = case shown="True" w481 {
          tunnel: w484 -> [w489 _]
          tunnel: [w487 FALSE ("Discard?")] -> w480
          tunnel: [w487 TRUE ("Discard?")] -> w479
          tunnel: w478 -> [w486 _]
          tunnel: w477 -> [w485 _]
          frame False {
            w487 = TRUE ("Discard?")
            n188 = case shown="True" w485 {
              tunnel: [cluster{"State":string}[] [{"State"="Save_PS_Config"}, {"State"="Write_PS_INI"}, {"State"="Close_GUI"}] cluster{"State":string}[] [{"State"="Save_PS_Config"}, {"State"="Write_PS_INI"}, {"State"="PS_Off"}, {"State"="Close_GUI"}]] -> w488
              frame False {
              }
              frame True {
              }
            }
            n189 = call "Queue Add Events to Back.vi"("Queue In"=w489, "State Array"=w488, "Error In"=w486) -> ()  [unwired: 11 in, 2 out]
          }
          frame True {
            n190 = One Button Dialog(message="Power Supply is Locked!!\nPower OFF PS before exiting") -> ()  [unwired: 1 in, 1 out]
          }
        }
        n191 = event-data("Discard?"=w479) -> ()  [unwired: 1 in, 1 out]
      }
    }
  }
  "Revision" <- "1.0.1" ("Revision")
